vi "Enable Output.vi"(8 "error in (no error)":errorcluster, 9 "Enable Output (F: Disable)":bool, 10 "Channel (1)":string="1", 11 "VISA resource name":refnum<visa-resource-name>) -> (0 "error out":errorcluster, 3 "VISA resource name out":refnum<visa-resource-name>)   [LabVIEW 2023, in "Keysight E36300 Series.lvlib"]
doc: "Enables or disables the specified output."
uses:
  Keysight E36300 Series.lvlib
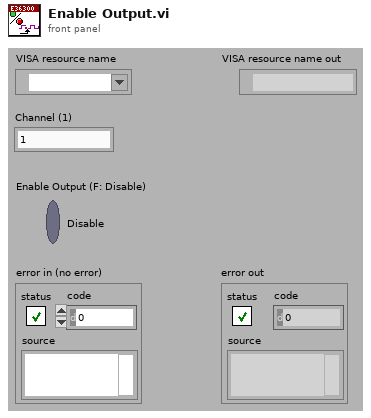
[diagram p1: front panel]
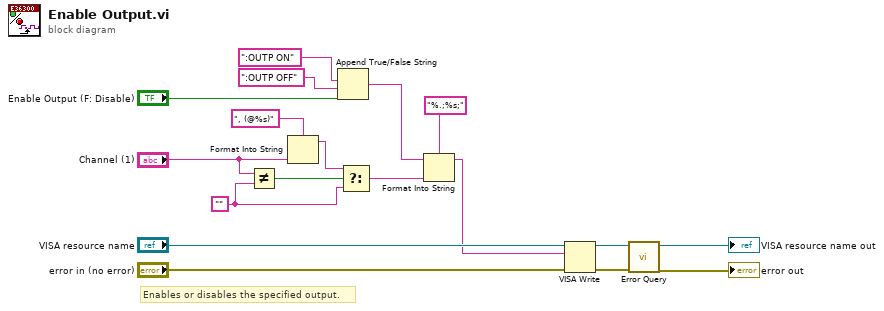
[diagram p0: block diagram]
diagram:
  w1 = ""
  # "Enables or disables the specified output."
  n1 = Not Equal?(x="Channel (1)", y=w1) -> (x != y?=w4:bool)
  n2 = Format Into String(format string=", (@%s)", "Channel (1)") -> (resulting string=w5:string)  [unwired: 2 in, 1 out]
  n3 = Append True/False String(1:"Enable Output (F: Disable)", 2:":OUTP OFF", 3:":OUTP ON") -> (0:w8:string)  [unwired: 1 in]
  n4 = Select(t=w5, s=w4, f=w1) -> (s? t:f=w2:string)
  n5 = Format Into String(format string="%.;%s;", initial string=w8, w2) -> (resulting string=w7:string)  [unwired: 1 in, 1 out]
  n6 = VISA Write(VISA resource name="VISA resource name", write buffer=w7, error in (no error)="error in (no error)") -> (VISA resource name out=w13:refnum<visa-resource-name>, error out=w12:errorcluster)  [unwired: 1 out]
  n7 = call "Error Query.vi"("error in (no error)"=w12, "VISA resource name"=w13) -> ("error out"=→"error out":errorcluster, "VISA resource name out"=→"VISA resource name out":refnum<visa-resource-name>)  [unwired: 6 in, 2 out]
